vi "replaceDateToken.vi"(8 "error in (no error)":errorcluster, 10 "Querry In":string, 11 "Goal in":refnum<class "Goal.lvclass">) -> (0 "error out":errorcluster, 2 "Query Out":string, 3 "Goal out":refnum<class "Goal.lvclass">)   [LabVIEW 2018, in "Goal.lvclass"]
uses:
  Goal.lvclass
  Goal.lvclass/Goal.ctl
  WhichMonth/WhichMonth.lvclass
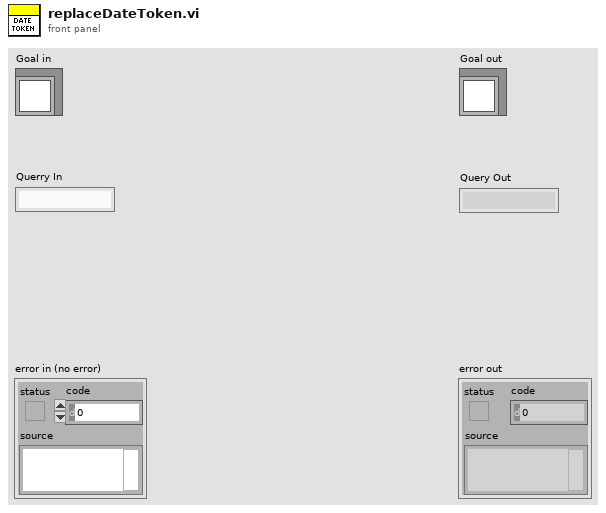
[diagram p1: front panel]
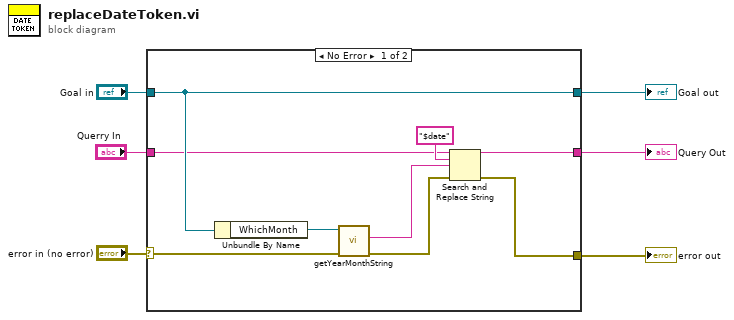
[diagram p0: block diagram]
diagram:
  n1 = case shown="No Error" "error in (no error)" {
    selector: "error in (no error)" -> [w11 w17]
    tunnel: [w9 w17] -> w5
    tunnel: [w14 w16] -> w3
    tunnel: "Goal in" -> [w14 w16]
    tunnel: [w10 _] -> w2
    tunnel: "Querry In" -> [w7 _]
    frame No Error {
      n2 = Unbundle By Name(w14) -> ("WhichMonth"=w13:refnum<class "WhichMonth.lvclass">)
      n3 = call "getYearMonthString.vi"("error in (no error)"=w11, "WhichMonth in"=w13) -> ("error out"=w8:errorcluster, "Year-Month"=w12:string)  [unwired: 7 in, 1 out]
      n4 = Search and Replace String(input string=w7, search string="$date", replace string=w12, error in=w8) -> (result string=w10:string, error out=w9:errorcluster)  [unwired: 4 in, 2 out]
    }
    frame Error {
    }
  }
  "error out" <- w5
  "Goal out" <- w3
  "Query Out" <- w2
